vi "Keep_Track_of_Volume.vi"() -> ()   [LabVIEW 2016]
uses:
  Labjack/ValveGlobals.vi
  <userlib>/_OpenG.lib/array/array.llb/Index 1D Array Elements (String)__ogtk.vi
panel:
  out "Pressure Changes (mbar)":dbl[](array[numeric])
  out "Volume (uL)":dbl[](array[numeric])
  out "Current Valve Flow Rate":dbl[](array[numeric])
  out "Pressure Groups":i32[](array[numeric])
  out "Pressure Group":u8[](array[numeric])=[3, 3, 3, 3, 4, 4, 4, 4]
  out "Valves in Use":string[](array[string])
  in  "Ctr Odor Valve":u16(ring)=14 items=["A1", "A2", "A3", "A4", "B1", "B2", "B3", "B4", "B5", "B6", "B7", "B8", "A5", "A6", "A7", "A8"]
  in  "Ctr Water Valve":u16(ring)=15 items=["A1", "A2", "A3", "A4", "B1", "B2", "B3", "B4", "B5", "B6", "B7", "B8", "A5", "A6", "A7", "A8"]
  in  "Valves Used":u16[](array[ring])=[0, 1, 2, 3, 8, 9, 10, 11] items=["A1", "A2", "A3", "A4", "B1", "B2", "B3", "B4", "B5", "B6", "B7", "B8"]
  out "flow meter 1 (ul/min)":dbl
  in  "stop":bool
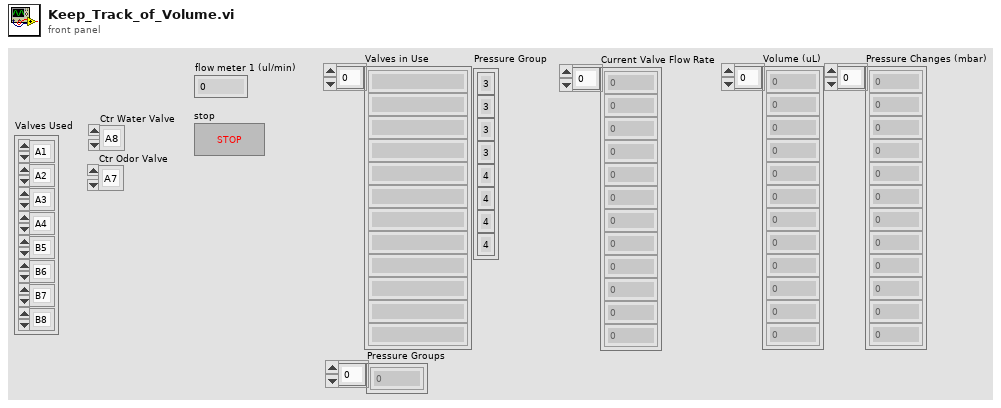
[diagram p1: front panel]
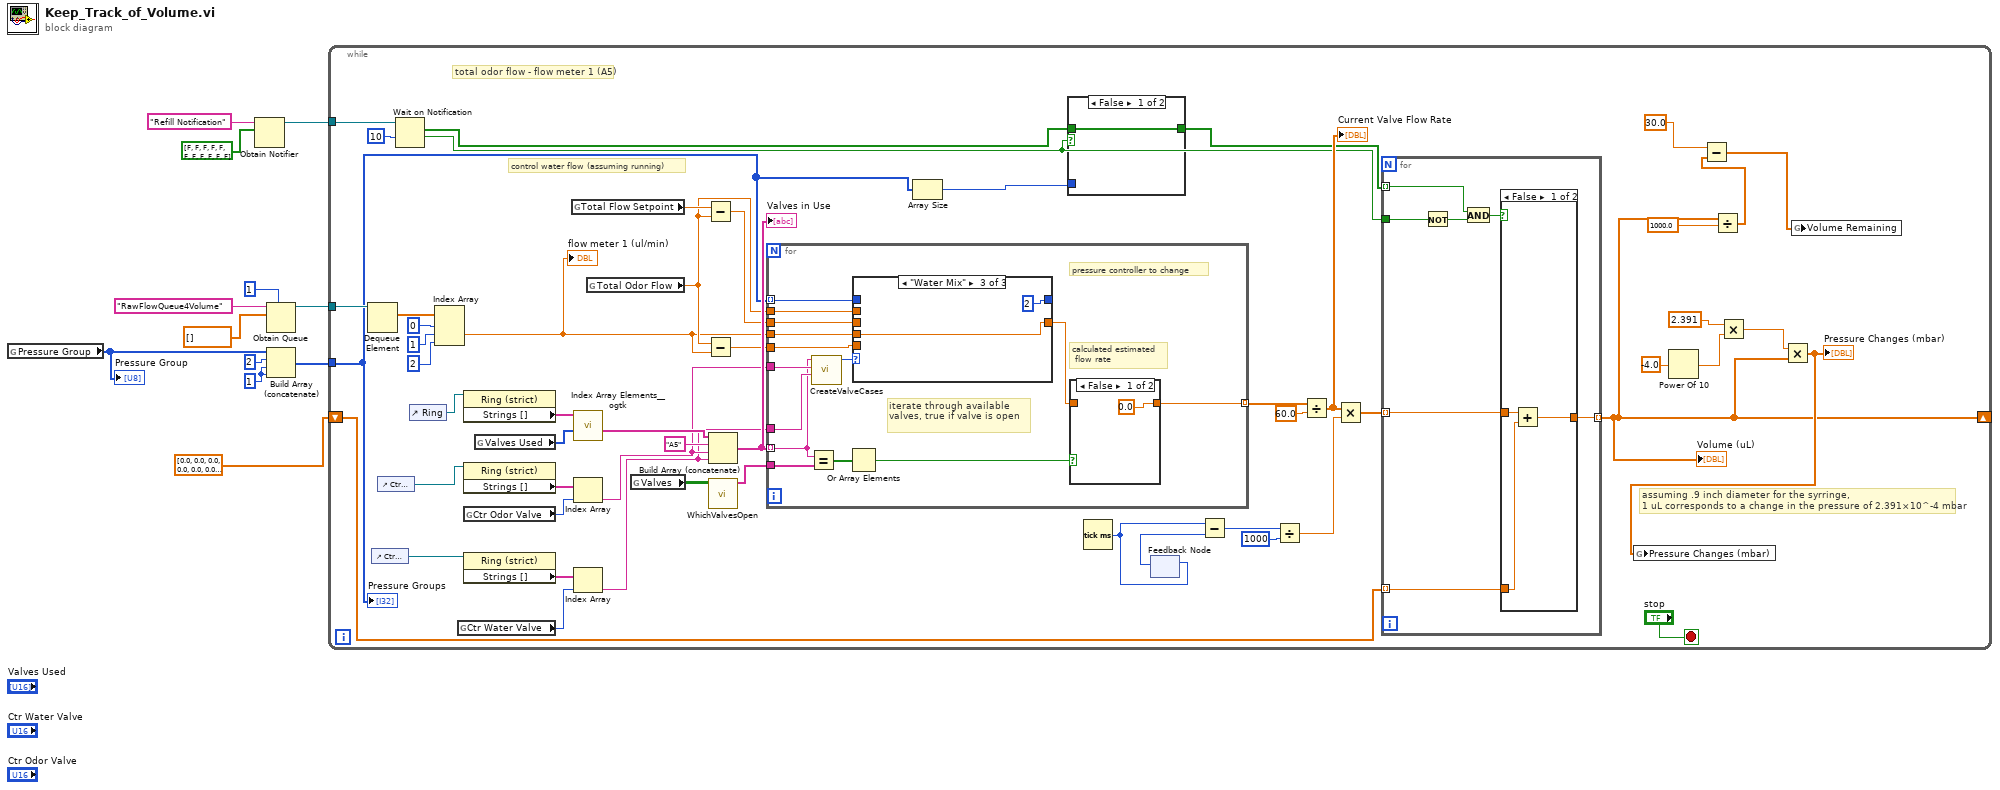
[diagram p0: block diagram]
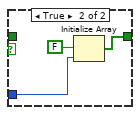
[diagram p2: hidden frame]
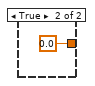
[diagram p3: hidden frame]
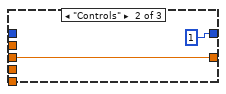
[diagram p5: hidden frame]
diagram:
  w9 = 1
  n1 = global read "ValveGlobals.vi" "Pressure Group"() -> (w7:u8[])
  "Pressure Group" <- w7
  n2 = Obtain Notifier(name (unnamed)="Refill Notification", notification data type=bool[] [FALSE, FALSE, FALSE, FALSE, FALSE, FALSE, FALSE, FALSE, FALSE, FALSE, FALSE] ("Refill!")) -> (notifier out=w3:refnum<notifier>)  [unwired: 2 in, 2 out]
  n3 = Obtain Queue(max queue size (-1, unlimited)=1, name (unnamed)="RawFlowQueue4Volume", element data type=dbl[] [] ("appended array")) -> (queue out=w10:refnum<queue>)  [unwired: 2 in, 2 out]
  n4 = Build Array (concatenate)(w7, 2, w9, w9) -> (w6:i32[])
  n5 = while {
    tunnel: w10 -> [w65]
    tunnel: w6 -> [w25]
    tunnel: w3 -> [w38]
    shift-right: [w16] -> _
    shift-left: dbl[] [0.0, 0.0, 0.0, 0.0, 0.0, 0.0, 0.0, 0.0, 0.0, 0.0, 0.0] ("Current Valve Flow Rate 2") -> [w30]
    stop <- "stop" stop-if-true
    # "assuming .9 inch diameter for the syrringe, \n1 uL corresponds to a change in the pressure of 2.391×10^-4 mbar"
    # "control water flow (assuming running)"
    # "total odor flow - flow meter 1 (A5)"
    n6 = Dequeue Element(queue=w65) -> (element=w64:dbl[])  [unwired: 2 in, 3 out]
    n7 = control-ref of="Ctr Water Valve"() -> (w56:refnum<vi>)
    n8 = control-ref of="Ctr Odor Valve"() -> (w55:refnum<vi>)
    n9 = Wait on Notification(notifier=w38, timeout in ms (-1)=10) -> (notification=w27:bool[], timed out?=w28:bool)  [unwired: 2 in, 2 out]
    n10 = control-ref of="Ring"() -> (w59:refnum<vi>)
    n11 = Index Array(array=w64, index #1=0 ("index"), index #2=1 ("index"), index #3=2 ("index")) -> (element #2=w40:dbl)  [unwired: 2 out]
    "flow meter 1 (ul/min)" <- w40
    n12 = global read "ValveGlobals.vi" "Ctr Water Valve"() -> (w51:u16)
    n13 = property class="Ring (strict)"(reference=w59) -> ("Strings []"=w58:string[])  [unwired: 1 in, 2 out]
    n14 = property class="Ring (strict)"(reference=w55) -> ("Strings []"=w54:string[])  [unwired: 1 in, 2 out]
    n15 = global read "ValveGlobals.vi" "Ctr Odor Valve"() -> (w53:u16)
    n16 = property class="Ring (strict)"(reference=w56) -> ("Strings []"=w52:string[])  [unwired: 1 in, 2 out]
    n17 = global read "ValveGlobals.vi" "Valves Used"() -> (w57:u16[])
    n18 = global read "ValveGlobals.vi" "Total Flow Setpoint"() -> (w42:dbl)
    n19 = call-poly <userlib>:"Index Array Elements__ogtk.vi"("indices"=w57, "array"=w58) -> ("elements"=w50:string[])  [unwired: 9 in]
    n20 = Index Array(array=w54, index=w53) -> (element=w46:string)
    n21 = Index Array(array=w52, index=w51) -> (element=w45:string)
    n22 = global read "ValveGlobals.vi" "Total Odor Flow"() -> (w41:dbl)
    n23 = global read "ValveGlobals.vi" "Valves"() -> (w60:bool[][])
    n24 = Subtract(x=w42, y=w41) -> (x-y=w44:dbl)
    n25 = Subtract(x=w41, y=w40) -> (x-y=w43:dbl)
    n26 = Build Array (concatenate)(w50, "A5", w46, w45) -> (w47:string[])
    "Valves in Use" <- w47
    n27 = call "WhichValvesOpen.vi"("Valves"=w60) -> ("appended array"=w48:string[])  [unwired: 10 in]
    n28 = for {
      tunnel: w48 -> [w95]
      tunnel: w47 -> [w82] mode=indexing
      tunnel: w46 -> [w92]
      tunnel: w45 -> [w89]
      tunnel: w25 -> [w90] mode=indexing
      tunnel: w41 -> [w88]
      tunnel: w44 -> [w87]
      tunnel: w43 -> [w86]
      tunnel: w40 -> [w85]
      tunnel: [w83] -> w36 mode=indexing
      # "calculated estimated\n flow rate"
      # "pressure controller to change"
      # "iterate through available valves, true if valve is open"
      n29 = Equal?(x=w82, y=w95) -> (x = y?=w94:bool[])
      n30 = call "CreateValveCases.vi"("Ctr Water Valve"=w89, "Ctr Odor Valve"=w92, "Valve In"=w82) -> ("Case"=w91:enum16{"Odors", "Controls", "Water Mix"})  [unwired: 8 in]
      n31 = Or Array Elements(Boolean array=w94) -> (logical OR=w93:bool)
      n32 = case shown="\"Water Mix\"" w91 {
        tunnel: w90 -> [w97 _ _]
        tunnel: [w97 1 ("Numeric") 2 ("Numeric")] -> _
        tunnel: w88 -> [_ _ _]
        tunnel: w87 -> [_ w99 _]
        tunnel: [w96 w99 w100] -> w84
        tunnel: w86 -> [w96 _ _]
        tunnel: w85 -> [_ _ w100]
        frame "Odors" {
          # "Odor part of odor flow"
        }
        frame "Controls" {
        }
        frame "Water Mix" {
        }
      }
      n33 = case shown="False" w93 {
        tunnel: w84 -> [_ w103]
        tunnel: [0.0 ("Flow-Rate") w103] -> w83
        frame False {
        }
        frame True {
        }
      }
    }
    n34 = Array Size(array=w25) -> (size(s)=w24:i32)
    n35 = case shown="False" w28 {
      tunnel: w27 -> [w67 _]
      tunnel: [w67 w68] -> w26
      tunnel: w24 -> [_ w70]
      frame False {
      }
      frame True {
        n36 = Initialize Array(FALSE, w70) -> (w68:bool[])
      }
    }
    n37 = Tick Count (ms)() -> (millisecond timer value=w19:u32)
    n38 = feedback-in #1(w19) -> ()
    n39 = feedback #1() -> (w37:u32)  [unwired: 1 in]
    n40 = Subtract(x=w19, y=w37) -> (x-y=w33:u32)
    n41 = Divide(x=w33, y=u32 1000) -> (x/y=w31:dbl)
    n42 = Divide(x=w36, y=60.0) -> (x/y=w34:dbl[])
    "Current Valve Flow Rate" <- w34
    n43 = Multiply(x=w34, y=w31) -> (x*y=w29:dbl[])
    n44 = for {
      tunnel: w26 -> [w75] mode=indexing
      tunnel: w28 -> [w77]
      tunnel: w29 -> [w73] mode=indexing
      tunnel: [w72] -> w16 mode=indexing
      tunnel: w30 -> [w71] mode=indexing
      n45 = Not(x=w77) -> (.not. x?=w76:bool)
      n46 = And(x=w75, y=w76) -> (x .and. y?=w74:bool)
      n47 = case shown="False" w74 {
        tunnel: w73 -> [w79 _]
        tunnel: w71 -> [w80 _]
        tunnel: [w78 0.0] -> w72
        frame False {
          n48 = Add(x=w79, y=w80) -> (x+y=w78:dbl)
        }
        frame True {
        }
      }
    }
    "Volume (uL)" <- w16
    n49 = Power Of 10(x=-4.0) -> (10^x=w21:dbl)
    n50 = Divide(x=w16, y=1000.0) -> (x/y=w14:dbl[])
    n51 = Subtract(x=30.0, y=w14) -> (x-y=w13:dbl[])
    n52 = Multiply(x=2.391, y=w21) -> (x*y=w20:dbl)
    n53 = Multiply(x=w20, y=w16) -> (x*y=w18:dbl[])
    "Pressure Changes (mbar)" <- w18
    n54 = global write "ValveGlobals.vi" "Pressure Changes (mbar)"(w18) -> ()
    n55 = global write "ValveGlobals.vi" "Volume Remaining"(w13) -> ()
    "Pressure Groups" <- w25
  }
